vi "Resize Panel to Pane.vi"(8 "error in (no error)":errorcluster, 10 "Apply Recursively? (F)":bool, 11 "IViewManager In":refnum<class "IViewManager.lvclass">) -> (0 "error out":errorcluster, 3 "IViewManager Out":refnum<class "IViewManager.lvclass">)   [LabVIEW 2017, in "IViewManager.lvlib" / "IViewManager.lvclass"]
doc: "<License>\nCopyright © 2017 Composed Systems, LLC | All rights reserved\nwww.composed.io\n\nAuthor: Ethan Stern <ethan.stern@composed.io>\n\nThis software is provided \"AS IS\" WITHOUT WARRANTIES, either express or implied, AND IS FOR EDUCATIONAL PURPOSES ONLY.\n</License>"
uses:
  <vilib>/gpm_packages/@cs/mva-viewable/Source/IViewManager/IViewManager/IViewManager.lvclass
  <vilib>/gpm_packages/@cs/mva-viewable/Source/IViewManager/IViewManager/IViewManager.lvclass/IViewManager.ctl
  <vilib>/gpm_packages/@cs/mva-viewable/Source/IViewable/IViewable Messages/Resize Panel to Pane Msg/Resize Panel to Pane Msg.lvclass/Resize Panel to Pane Msg.ctl
  <vilib>/ActorFramework/Message Enqueuer/Message Enqueuer.lvclass/Message Enqueuer.ctl
  <vilib>/ActorFramework/Message Enqueuer/Enqueue.vi
  <vilib>/gpm_packages/@cs/mva-viewable/Source/IViewable/IViewable Messages/Resize Panel to Pane Msg/Resize Panel to Pane Msg.lvclass
  C:/Program Files/National Instruments/LabVIEW 2017/vi.lib/ActorFramework/Message/Message.lvclass
  <vilib>/ActorFramework/Message Priority Queue/Priority Enqueue.vi
  <vilib>/gpm_packages/@cs/mva-viewable/Source/IViewable/IViewable/IViewable.lvclass
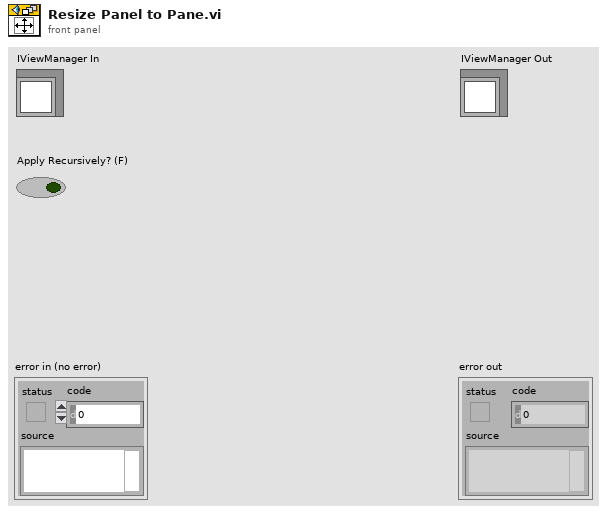
[diagram p1: front panel]
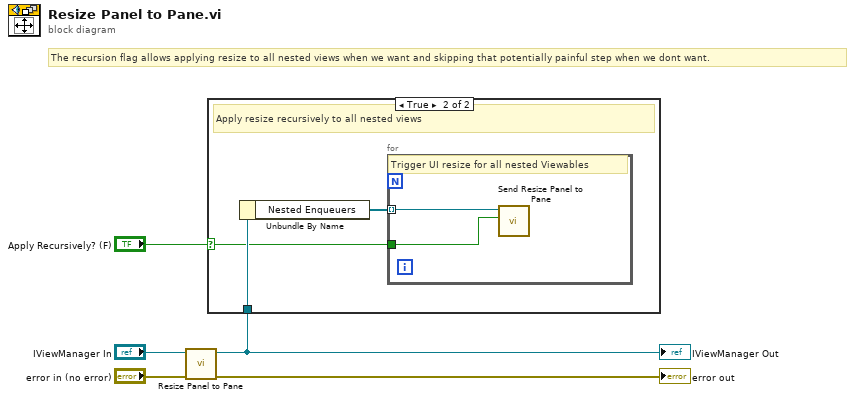
[diagram p0: block diagram]
diagram:
  # "The recursion flag allows applying resize to all nested views when we want and skipping that potentially painful step when we dont want."
  n1 = call-parent "Resize Panel to Pane.vi"("error in (no error)"="error in (no error)", "IViewable In"="IViewManager In") -> ("error out"=→"error out":errorcluster, "IViewable Out"=w2:refnum<class "IViewManager.lvclass">)  [unwired: 8 in]
  "IViewManager Out" <- w2
  n2 = case shown="True" "Apply Recursively? (F)" {
    selector: "Apply Recursively? (F)" -> [_ w6]
    tunnel: w2 -> [_ w8]
    frame False {
      # "Do not apply resize to any nested views"
    }
    frame True {
      # "Apply resize recursively to all nested views"
      n3 = Unbundle By Name(w8) -> ("Nested Enqueuers"=w7:refnum<class "Message Enqueuer.lvclass">[])
      n4 = for {
        tunnel: w7 -> [w10] mode=indexing
        tunnel: w6 -> [w9]
        # "Trigger UI resize for all nested Viewables"
        n5 = call <vilib>:"Send Resize Panel to Pane.vi"("Apply Recursively? (F)"=w9, "Message Enqueuer"=w10) -> ()  [unwired: 8 in, 2 out]
      }
    }
  }
